vi "widgets.vi"(7 "LabVIEW Web Service Request":refnum<class "Web Request.lvclass">, 10 "laboratory_id":string, 11 "context_id":string) -> (3 "widgets":cluster{"name":string, "description":string}[](array[cluster]))   [LabVIEW 2013]
uses:
  <vilib>/wsapi/Web Request.lvclass
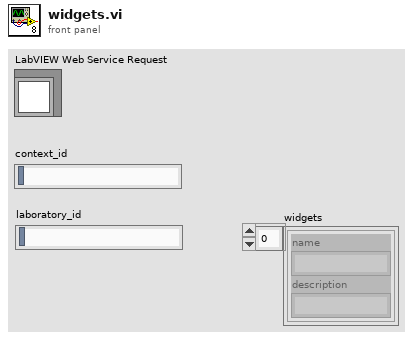
[diagram p1: front panel]
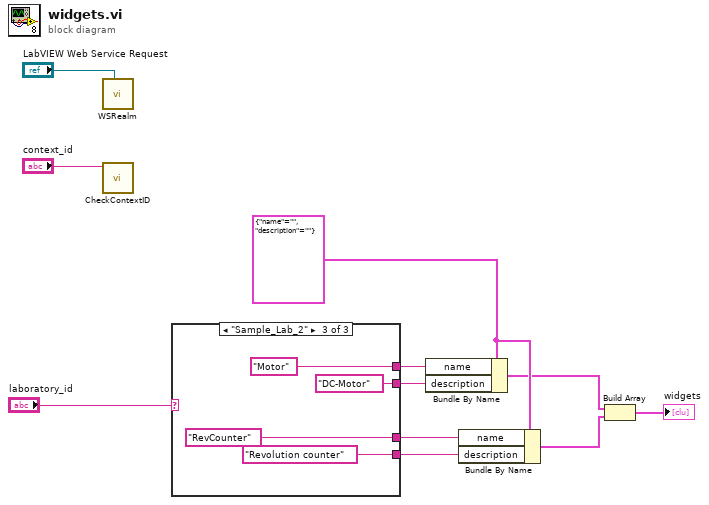
[diagram p0: block diagram]
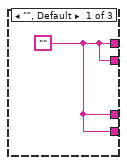
[diagram p2: hidden frame]
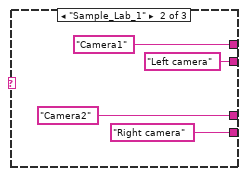
[diagram p3: hidden frame]
diagram:
  w9 = cluster{"name":string, "description":string} {"name"="", "description"=""}
  n1 = call "WSRealm.vi"("LabVIEW Web Service Request"="LabVIEW Web Service Request") -> ()  [unwired: 11 in]
  n2 = call "CheckContextID.vi"("context_id"="context_id") -> ()  [unwired: 10 in, 1 out]
  n3 = case shown="\"Sample_Lab_2\"" "laboratory_id" {
    tunnel: [w12 "Camera1" ("name") "Motor" ("name")] -> w7
    tunnel: [w12 "Left camera" "DC-Motor"] -> w6
    tunnel: [w12 "Camera2" ("name") "RevCounter" ("name")] -> w5
    tunnel: [w12 "Right camera" "Revolution counter"] -> w4
    frame "", Default {
      w12 = ""
    }
    frame "Sample_Lab_1" {
    }
    frame "Sample_Lab_2" {
    }
  }
  n4 = Bundle By Name(cluster=w9, "name"=w7, "description"=w6) -> (w3:cluster{"name":string, "description":string})
  n5 = Bundle By Name(cluster=w9, "name"=w5, "description"=w4) -> (w2:cluster{"name":string, "description":string})
  n6 = Build Array(w3, w2) -> (→"widgets":cluster{"name":string, "description":string}[])
